vi "数据写入.vi"(9 "CAN通道":u8, 10 "ID":u32, 11 "簇":T1) -> ()   [LabVIEW 2021]
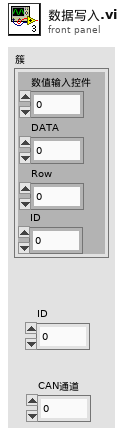
[diagram p1: front panel]
types:
  T1 = cluster{"数值输入控件":u16, "DATA":u32, "Row":i32, "ID":i32}
  T2 = cluster{"ID":u32, "MSGTYPE":u8, "LEN":u8, i32, i32, u8, u8, u8, u8, i32, i32}
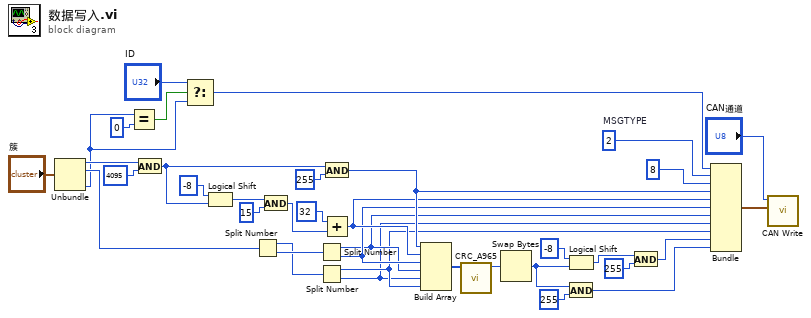
[diagram p0: block diagram]
diagram:
  w37 = u8 2  # MSGTYPE
  n1 = Unbundle("簇") -> ("数值输入控件"=w16:u16, "DATA"=w14:u32, "ID"=w2:i32)  [unwired: 1 out]
  n2 = Equal?(x=w2, y=0) -> (x = y?=w4:bool)
  n3 = And(x=w16, y=4095) -> (x .and. y?=w22:i32)
  n4 = Select(t="ID", s=w4, f=w2) -> (s? t:f=w1:u32)
  n5 = Logical Shift(y=i16 -8, x=w22) -> (x << y=w20:i32)
  n6 = Split Number(x=w14) -> (hi(x)=w12:u16, lo(x)=w13:u16)
  n7 = And(x=w20, y=15) -> (x .and. y?=w35:i32)
  n8 = Split Number(x=w13) -> (hi(x)=w23:u8, lo(x)=w24:u8)
  n9 = Split Number(x=w12) -> (hi(x)=w11:u8, lo(x)=w10:u8)
  n10 = And(x=w22, y=255) -> (x .and. y?=w26:i32)
  n11 = Add(x=u8 32 ("DATA[1]"), y=w35) -> (x+y=w25:i32)
  n12 = Build Array(w26, w25, w24, w23, w10, w11) -> (w7:i32[])
  n13 = call "CRC_A965 .vi"("U8"=w7) -> ("CRC-16"=w6:u16)  [unwired: 10 in]
  n14 = Swap Bytes(anything=w6) -> (byte swapped=w18:u16)
  n15 = Logical Shift(y=i16 -8, x=w18) -> (x << y=w17:u16)
  n16 = And(x=w18, y=255) -> (x .and. y?=w28:i32)
  n17 = And(x=w17, y=255) -> (x .and. y?=w27:i32)
  n18 = Bundle("ID"=w1, "MSGTYPE"=w37, "LEN"=u8 8, w26, w25, w24, w23, w10, w11, w27, w28) -> (w8:T2)  [unwired: 1 in]
  n19 = call "CAN Write.vi"("MessageBuffer"=w8, "Channel"="CAN通道") -> ()  [unwired: 7 in, 3 out]
